vi "Sweep Parameters.vi"(8 "error in (no error)":errorcluster, 11 "VISA resource name":refnum<visa-resource-name>) -> (0 "error out":errorcluster, 1 "Span":dbl format="%^.3e", 2 "Center":dbl format="%^.3e", 3 "VISA resource name out":refnum<visa-resource-name>, 4 "Step":dbl format="%^.3e", 5 "Stop":dbl format="%^.3e", 6 "Number of points":i32, 7 "Start":dbl format="%^.3e")   [LabVIEW 2017, in "Agilent 4194.lvlib"]
doc: "This function outputs the sweep parameters data."
uses:
  Agilent 4194.lvlib
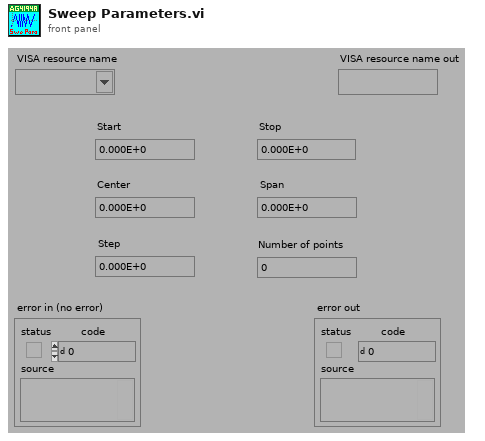
[diagram p1: front panel]
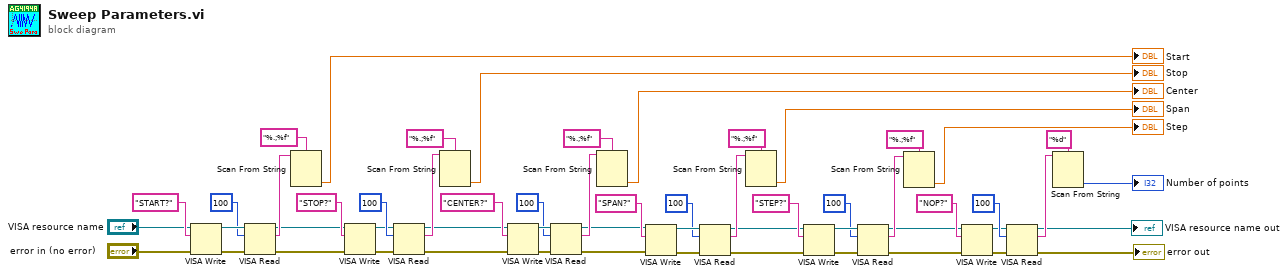
[diagram p0: block diagram]
diagram:
  n1 = VISA Write(VISA resource name="VISA resource name", write buffer="START?" ("write buffer (\"\")"), error in (no error)="error in (no error)") -> (VISA resource name out=w36:refnum<visa-resource-name>, error out=w37:errorcluster)  [unwired: 1 out]
  n2 = VISA Read(VISA resource name=w36, byte count=u32 100 ("byte count (0)"), error in (no error)=w37) -> (VISA resource name out=w21:refnum<visa-resource-name>, read buffer=w33:string, error out=w20:errorcluster)  [unwired: 1 out]
  n3 = Scan From String(format string="%.;%f", input string=w33) -> (output 1=→"Start":dbl)  [unwired: 3 in, 3 out]
  n4 = VISA Write(VISA resource name=w21, write buffer="STOP?" ("write buffer (\"\")"), error in (no error)=w20) -> (VISA resource name out=w29:refnum<visa-resource-name>, error out=w28:errorcluster)  [unwired: 1 out]
  n5 = VISA Read(VISA resource name=w29, byte count=u32 100 ("byte count (0)"), error in (no error)=w28) -> (VISA resource name out=w19:refnum<visa-resource-name>, read buffer=w31:string, error out=w18:errorcluster)  [unwired: 1 out]
  n6 = Scan From String(format string="%.;%f", input string=w31) -> (output 1=→"Stop":dbl)  [unwired: 3 in, 3 out]
  n7 = VISA Write(VISA resource name=w19, write buffer="CENTER?" ("write buffer (\"\")"), error in (no error)=w18) -> (VISA resource name out=w26:refnum<visa-resource-name>, error out=w27:errorcluster)  [unwired: 1 out]
  n8 = VISA Read(VISA resource name=w26, byte count=u32 100 ("byte count (0)"), error in (no error)=w27) -> (VISA resource name out=w15:refnum<visa-resource-name>, read buffer=w24:string, error out=w14:errorcluster)  [unwired: 1 out]
  n9 = Scan From String(format string="%.;%f", input string=w24) -> (output 1=→"Center":dbl)  [unwired: 3 in, 3 out]
  n10 = VISA Write(VISA resource name=w15, write buffer="SPAN?" ("write buffer (\"\")"), error in (no error)=w14) -> (VISA resource name out=w41:refnum<visa-resource-name>, error out=w42:errorcluster)  [unwired: 1 out]
  n11 = VISA Read(VISA resource name=w41, byte count=u32 100 ("byte count (0)"), error in (no error)=w42) -> (VISA resource name out=w12:refnum<visa-resource-name>, read buffer=w38:string, error out=w13:errorcluster)  [unwired: 1 out]
  n12 = Scan From String(format string="%.;%f", input string=w38) -> (output 1=→"Span":dbl)  [unwired: 3 in, 3 out]
  n13 = VISA Write(VISA resource name=w12, write buffer="STEP?" ("write buffer (\"\")"), error in (no error)=w13) -> (VISA resource name out=w55:refnum<visa-resource-name>, error out=w56:errorcluster)  [unwired: 1 out]
  n14 = VISA Read(VISA resource name=w55, byte count=u32 100 ("byte count (0)"), error in (no error)=w56) -> (VISA resource name out=w45:refnum<visa-resource-name>, read buffer=w52:string, error out=w44:errorcluster)  [unwired: 1 out]
  n15 = Scan From String(format string="%.;%f", input string=w52) -> (output 1=→"Step":dbl)  [unwired: 3 in, 3 out]
  n16 = VISA Write(VISA resource name=w45, write buffer="NOP?" ("write buffer (\"\")"), error in (no error)=w44) -> (VISA resource name out=w48:refnum<visa-resource-name>, error out=w47:errorcluster)  [unwired: 1 out]
  n17 = VISA Read(VISA resource name=w48, byte count=u32 100 ("byte count (0)"), error in (no error)=w47) -> (VISA resource name out=→"VISA resource name out":refnum<visa-resource-name>, read buffer=w50:string, error out=→"error out":errorcluster)  [unwired: 1 out]
  n18 = Scan From String(format string="%d", input string=w50) -> (output 1=→"Number of points":i32)  [unwired: 3 in, 3 out]
